vi "Gui_Prrod_Cons.vi"() -> ()   [LabVIEW 2023]
uses:
  EnumTypeDef.ctl
  <vilib>/vision/Image Controls.llb/IMAQ Image.ctl
  Control 3.ctl
  Cluster1TypeDef.ctl
panel:
  out "Image":T1(plugin-control)
  in  "OK Button":bool
  in  "File Path":path
  in  "skala szaroœci 2":u8(slide) scale=0.0..100.0
  out "Image2":T1(plugin-control)
  in  "error in (no error) 2":errorcluster
  in  "error in (no error)":errorcluster
  in  "STOP":bool
  in  "START":bool
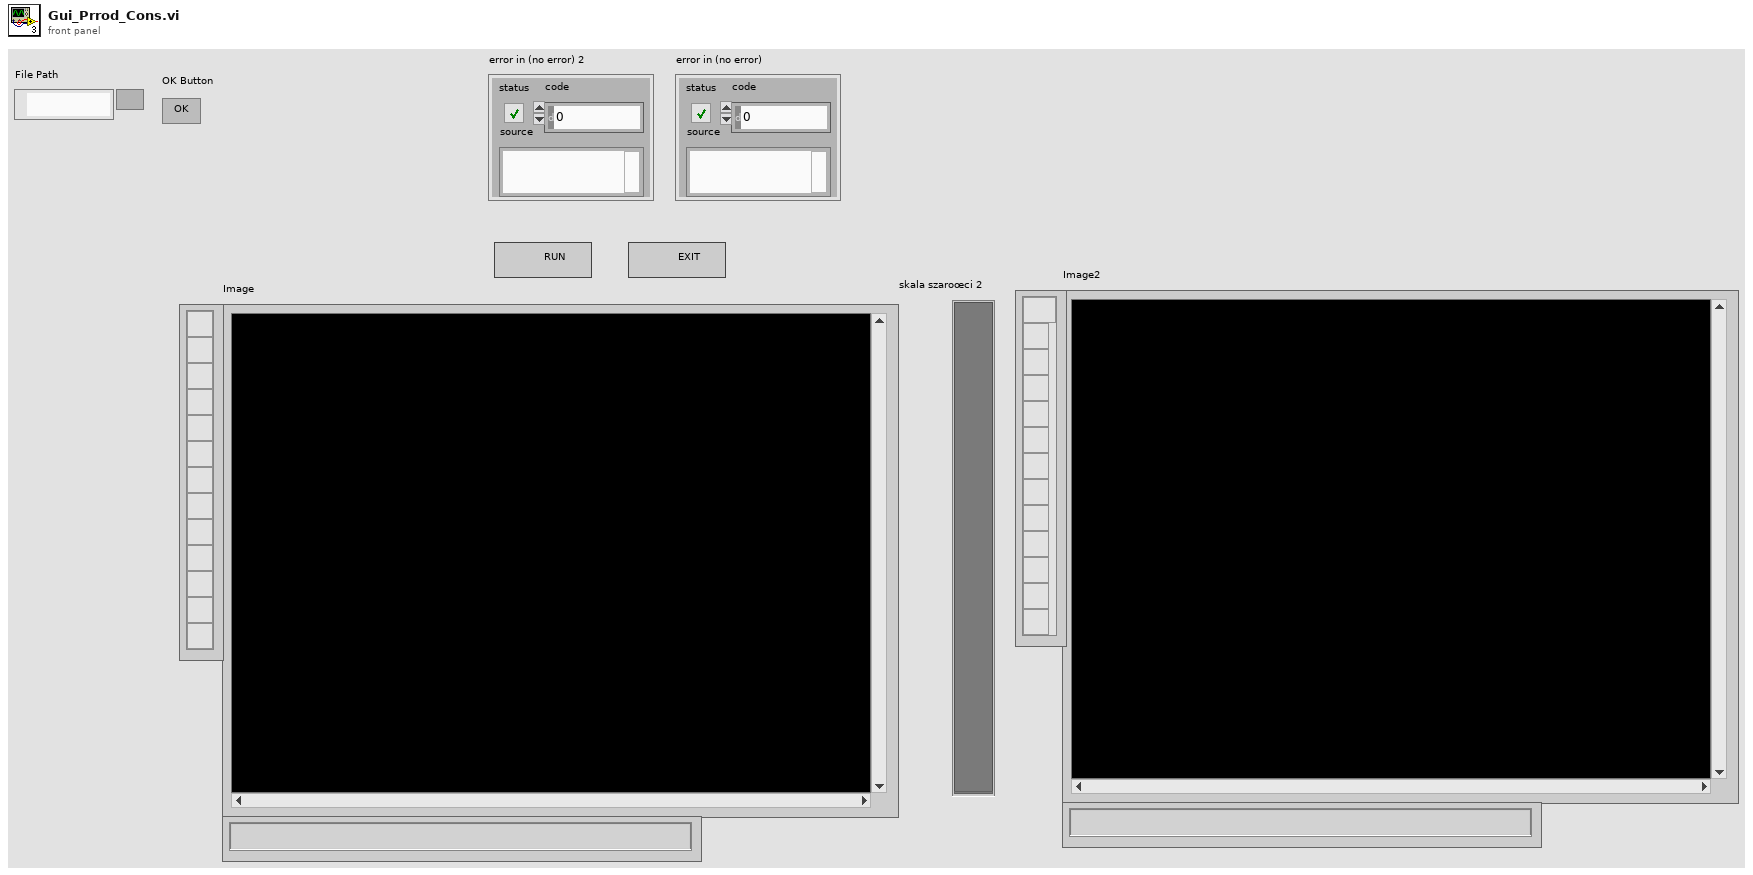
[diagram p1: front panel]
types:
  T1 = typedef "IMAQ Image.ctl" = refnum<image>
  T2 = typedef "Cluster1TypeDef.ctl" = cluster{"EditedImage":T1, "Enum":T3, "skala szaroœci 2":u8, "Data":variant, "Data2":variant}
  T3 = typedef "Control 3.ctl" = enum16{"Default", "PathLoaded", "RawImageLoaded", "LoadFile", "EditImage", "ImageEdited", "CloseAll"}
  T4 = cluster{"skala szaroœci 2":u8, "EditedImage":T1, "RawImage":T1, "Data":variant}
  T5 = typedef "EnumTypeDef.ctl" = enum16{"Initialize", "FilePathLoaded", "DisplayRaw", "EditImage", "ShutDown"}
  T6 = cluster{"skala szaroœci 2":u8, "Enum":T5, "RawImage":T1, "Data":variant}
  T7 = cluster{"EditedImage":T1, "Enum":T3, "skala szaroœci 2":u8, "Data":variant, "Data2":variant}
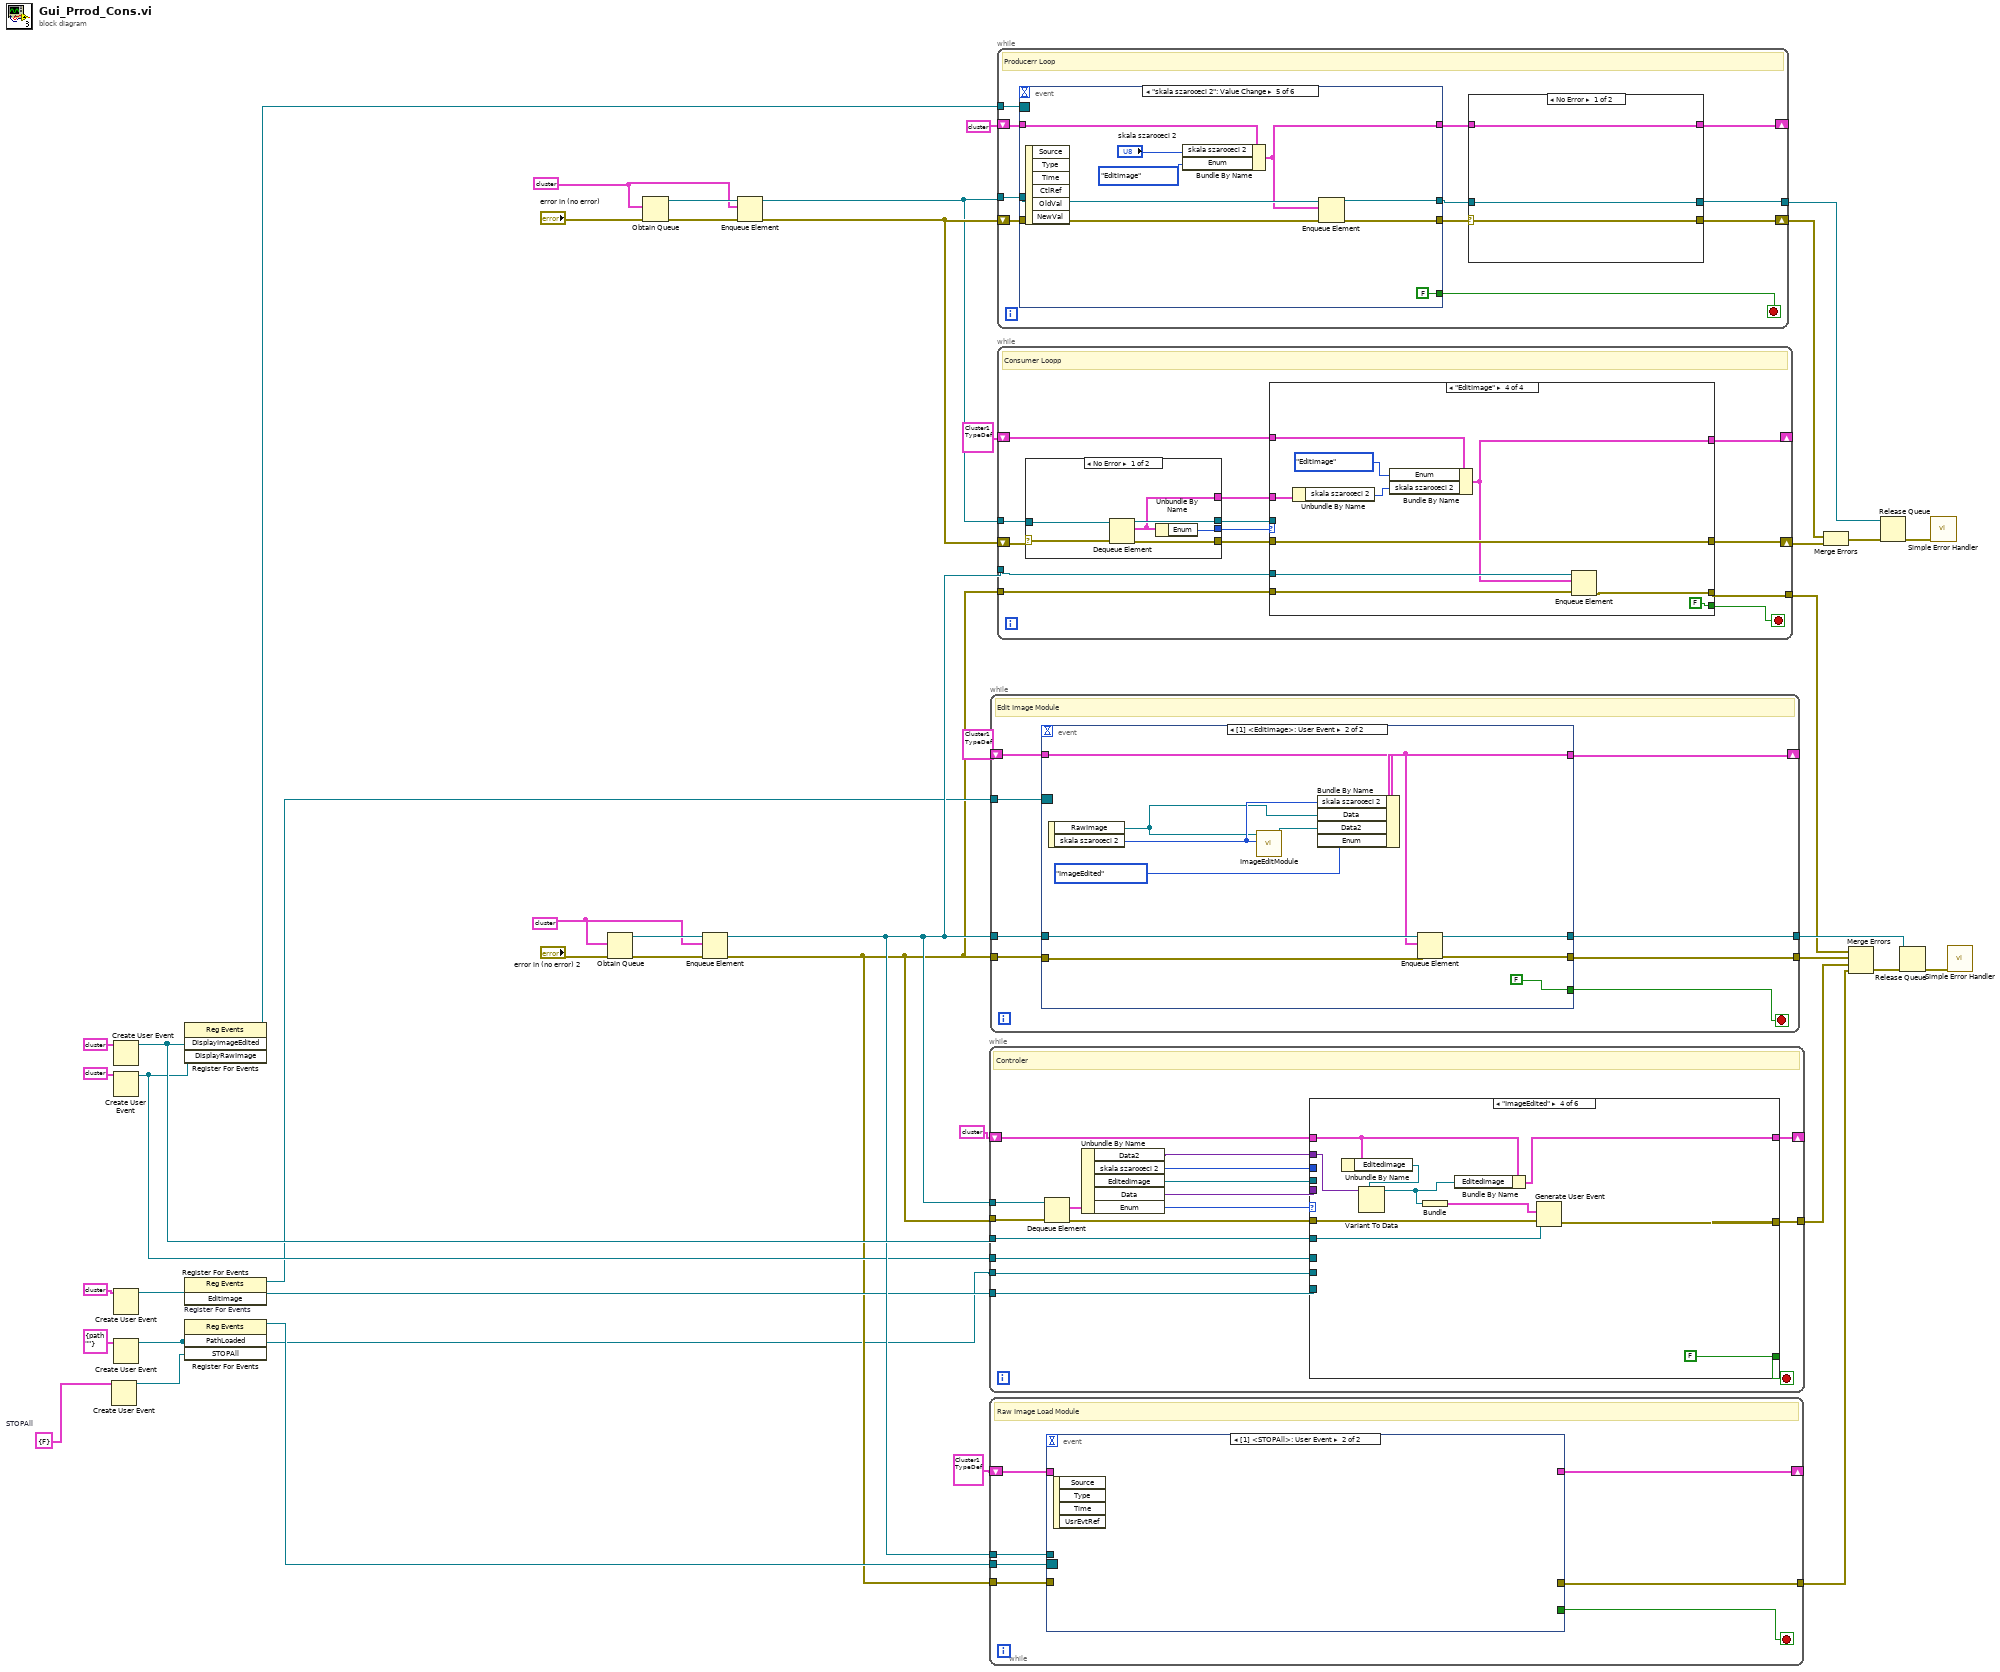
[diagram p0: block diagram]
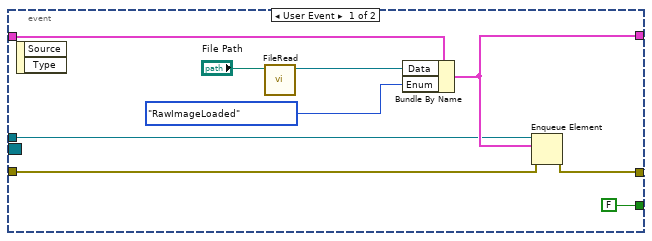
[diagram p2: hidden frame]
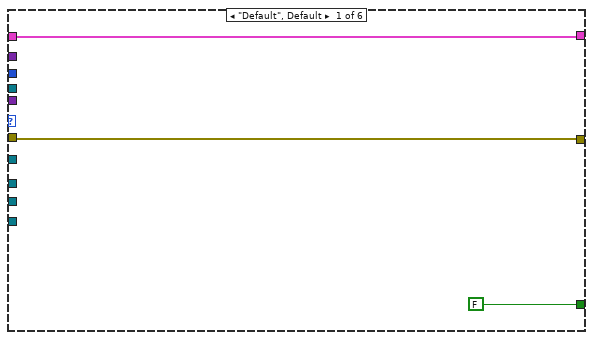
[diagram p3: hidden frame]
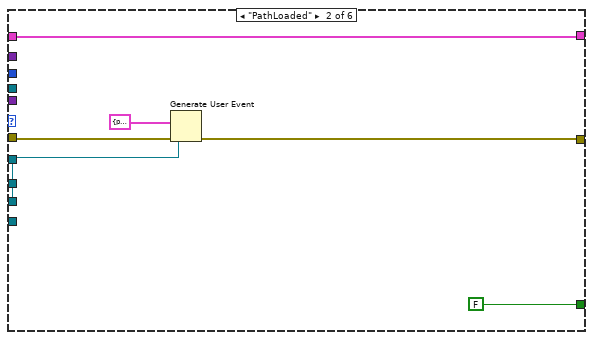
[diagram p4: hidden frame]
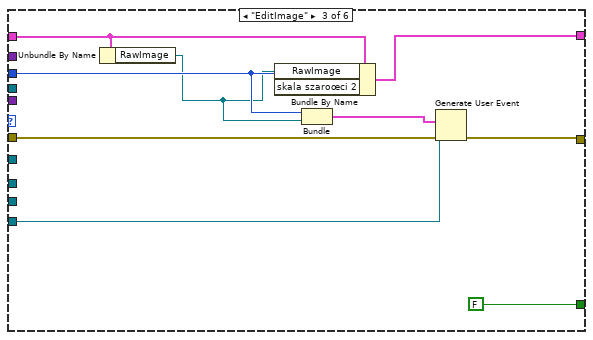
[diagram p5: hidden frame]
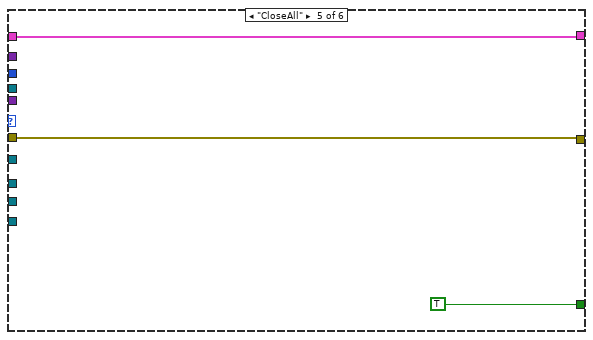
[diagram p6: hidden frame]
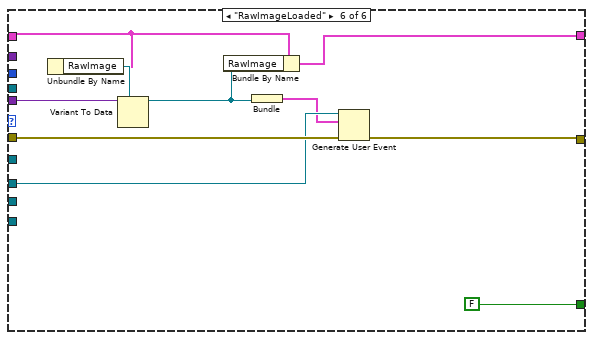
[diagram p7: hidden frame]
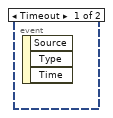
[diagram p8: hidden frame]
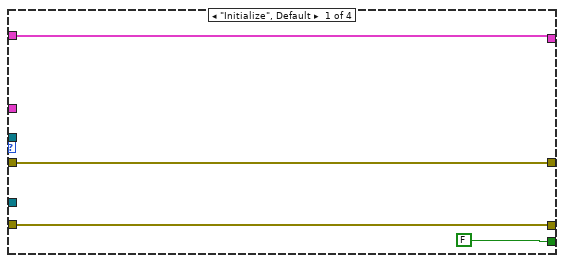
[diagram p9: hidden frame]
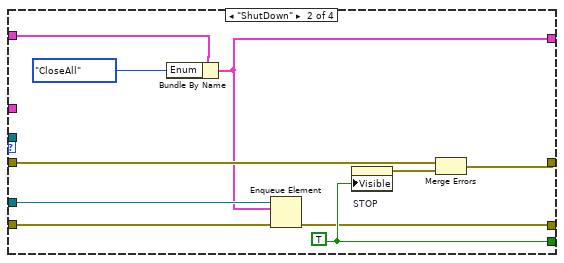
[diagram p10: hidden frame]
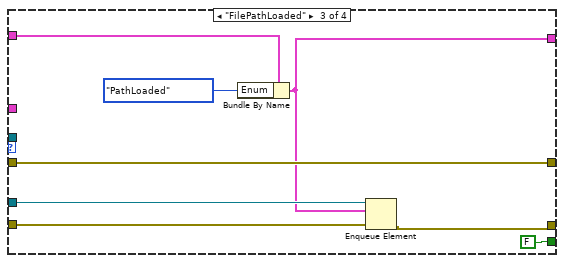
[diagram p11: hidden frame]
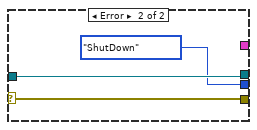
[diagram p12: hidden frame]
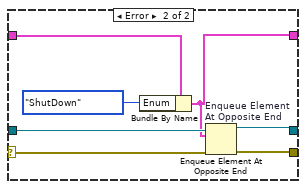
[diagram p13: hidden frame]
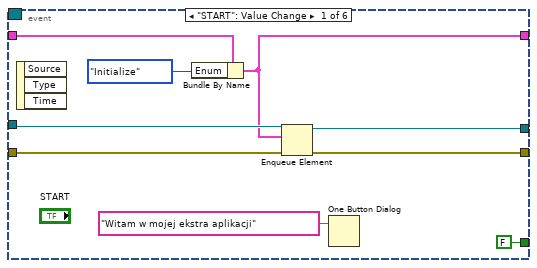
[diagram p14: hidden frame]
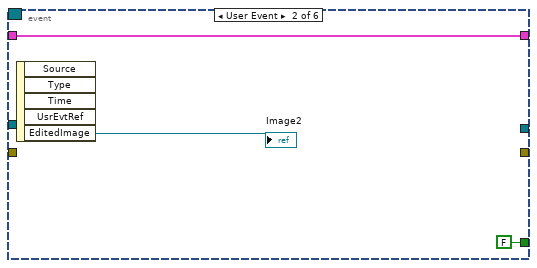
[diagram p15: hidden frame]
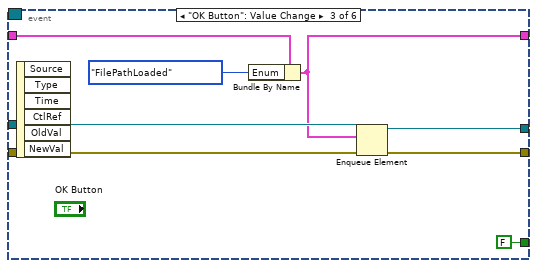
[diagram p16: hidden frame]
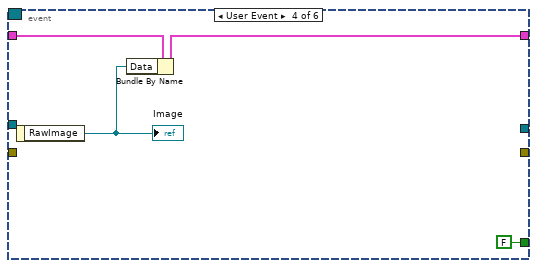
[diagram p17: hidden frame]
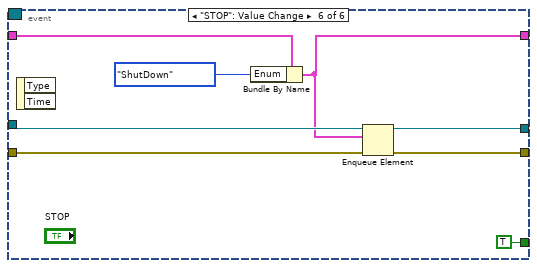
[diagram p18: hidden frame]
diagram:
  w2 = cluster{bool} {FALSE}  # STOPAll
  w16 = T6 {"skala szaroœci 2"=0, "Enum"=enum."Initialize", "RawImage"=refnum, "Data"=variant(refnum<image> refnum)} ("clusterSimple")
  w28 = T7 {"EditedImage"=refnum, "Enum"=enum."Default", "skala szaroœci 2"=0, "Data"=variant, "Data2"=variant(refnum<image> refnum)}
  n1 = Create User Event(user event datatype=w2) -> (user event=w1:refnum<user-event>)  [unwired: 1 in, 1 out]
  n2 = Create User Event(user event datatype=cluster{"EditedImage":T1} {"EditedImage"=refnum} ("DisplayImageEdited")) -> (user event=w25:refnum<user-event>)  [unwired: 1 in, 1 out]
  n3 = Create User Event(user event datatype=cluster{"RawImage":T1} {"RawImage"=refnum} ("DisplayRawImage")) -> (user event=w17:refnum<user-event>)  [unwired: 1 in, 1 out]
  n4 = Create User Event(user event datatype=cluster{"skala szaroœci 2":u8, "RawImage":T1} {"skala szaroœci 2"=0, "RawImage"=refnum} ("EditImage")) -> (user event=w13:refnum<user-event>)  [unwired: 1 in, 1 out]
  n5 = Create User Event(user event datatype=cluster{"File Path":path} {"File Path"=path ""} ("PathLoaded")) -> (user event=w7:refnum<user-event>)  [unwired: 1 in, 1 out]
  n6 = register-events(w25, w17) -> (reference out=w26:refnum<event-registration>)  [unwired: 2 in, 1 out]
  n7 = register-events(w13) -> (reference out=w10:refnum<event-registration>)  [unwired: 2 in, 1 out]
  n8 = register-events "Register For Events"(w7, w1) -> (reference out=w19:refnum<event-registration>)  [unwired: 2 in, 1 out]
  n9 = Obtain Queue(element data type=w28, error in (no error)="error in (no error) 2") -> (queue out=w30:refnum<queue>, error out=w31:errorcluster)  [unwired: 3 in, 1 out]
  n10 = Obtain Queue(element data type=w16, error in (no error)="error in (no error)") -> (queue out=w41:refnum<queue>, error out=w42:errorcluster)  [unwired: 3 in, 1 out]
  n11 = Enqueue Element(queue=w30, element=w28, error in (no error)=w31) -> (queue out=w18:refnum<queue>, error out=w9:errorcluster)  [unwired: 1 in, 1 out]
  n12 = Enqueue Element(queue=w41, element=w16, error in (no error)=w42) -> (queue out=w38:refnum<queue>, error out=w39:errorcluster)  [unwired: 1 in, 1 out]
  n13 = while {
    tunnel: w18 -> [w51]
    tunnel: w9 -> [w59]
    tunnel: w25 -> [w56]
    shift-right: [w54] -> _
    shift-left: T4 {"skala szaroœci 2"=0, "EditedImage"=refnum, "RawImage"=refnum, "Data"=variant(refnum<image> refnum)} ("EditImage") -> [w55]
    tunnel: [w52] -> w23
    tunnel: w7 -> [w50]
    tunnel: w17 -> [w49]
    tunnel: w13 -> [w48]
    stop <- w43 stop-if-true
    # "Controler"
    n14 = Dequeue Element(queue=w51, error in (no error)=w59) -> (element=w57:T7, error out=w53:errorcluster)  [unwired: 1 in, 2 out]
    n15 = Unbundle By Name(w57) -> ("Data2"=w44:variant, "skala szaroœci 2"=w45:u8, "EditedImage"=w46:T1, "Data"=w47:variant, "Enum"=w58:T3)
    n16 = case shown="\"ImageEdited\"" w58 {
      tunnel: w46 -> [_ _ _ _ _ _]
      tunnel: w56 -> [_ _ _ w87 _ _]
      tunnel: w55 -> [w62 w68 w71 w83 w88 w95]
      tunnel: [w62 w68 w74 w84 w88 w94] -> w54
      tunnel: w53 -> [w61 w67 w77 w86 w89 w100]
      tunnel: [w61 w66 w76 w85 w89 w99] -> w52
      tunnel: w50 -> [_ w65 _ _ _ _]
      tunnel: w49 -> [_ _ _ _ _ w98]
      tunnel: w48 -> [_ _ w75 _ _ _]
      tunnel: w47 -> [_ _ _ _ _ w97]
      tunnel: w45 -> [_ _ w73 _ _ _]
      tunnel: w44 -> [_ _ _ w79 _ _]
      tunnel: [FALSE FALSE FALSE FALSE TRUE FALSE] -> w43
      frame "Default", Default {
      }
      frame "PathLoaded" {
        n17 = Generate User Event(user event=w65, event data cluster=cluster{"File Path":path} {"File Path"=path ""} ("event data"), error in=w67) -> (error out=w66:errorcluster)  [unwired: 1 in, 1 out]
      }
      frame "EditImage" {
        n18 = Unbundle By Name(w71) -> ("RawImage"=w70:T1)
        n19 = Bundle By Name(cluster=w71, "RawImage"=w70, "skala szaroœci 2"=w73) -> (w74:T4)
        n20 = Bundle("skala szaroœci 2"=w73, "RawImage"=w70) -> (w72:cluster{"skala szaroœci 2":u8, "RawImage":T1})  [unwired: 1 in]
        n21 = Generate User Event(user event=w75, event data cluster=w72, error in=w77) -> (error out=w76:errorcluster)  [unwired: 1 in, 1 out]
      }
      frame "ImageEdited" {
        n22 = Unbundle By Name(w83) -> ("EditedImage"=w82:T1)
        n23 = Variant To Data(type=w82, Variant=w79) -> (data=w81:T1)  [unwired: 1 in, 1 out]
        n24 = Bundle("EditedImage"=w81) -> (w80:cluster{"EditedImage":T1})  [unwired: 1 in]
        n25 = Bundle By Name(cluster=w83, "EditedImage"=w81) -> (w84:T4)
        n26 = Generate User Event(user event=w87, event data cluster=w80, error in=w86) -> (error out=w85:errorcluster)  [unwired: 1 in, 1 out]
      }
      frame "CloseAll" {
      }
      frame "RawImageLoaded" {
        n27 = Unbundle By Name(w95) -> ("RawImage"=w96:T1)
        n28 = Variant To Data(type=w96, Variant=w97) -> (data=w93:T1)  [unwired: 1 in, 1 out]
        n29 = Bundle By Name(cluster=w95, "RawImage"=w93) -> (w94:T4)
        n30 = Bundle("RawImage"=w93) -> (w92:cluster{"RawImage":T1})  [unwired: 1 in]
        n31 = Generate User Event(user event=w98, event data cluster=w92, error in=w100) -> (error out=w99:errorcluster)  [unwired: 1 in, 1 out]
      }
    }
  }
  n32 = while {
    shift-right: [w102] -> _
    shift-left: T2 {"EditedImage"=refnum, "Enum"=enum."Default", "skala szaroœci 2"=0, "Data"=variant(refnum<image> refnum), "Data2"=variant(refnum<image> refnum)} ("Cluster") -> [w107]
    tunnel: w19 -> [w106]
    tunnel: w18 -> [w105]
    tunnel: w9 -> [w104]
    tunnel: [w103] -> w8
    stop <- w101 stop-if-true
    # "Raw Image Load Module"
    n33 = event shown="[1] <STOPAll>: User Event" {
      selector: w106 -> [_ _]
      dyn-events: _ -> [_ _]
      timeout: _ -> [_ _]
      tunnel: [w113 _] -> w102
      tunnel: w107 -> [w115 _]
      tunnel: w105 -> [w111 _]
      tunnel: w104 -> [w112 _]
      tunnel: [w110 _] -> w103
      tunnel: [FALSE _] -> w101
      event User Event {
        n34 = event-data() -> ()  [unwired: 1 in, 2 out]
        n35 = call "FileRead.vi"("File Path"="File Path") -> ("Image"=w109:T1)  [unwired: 10 in]
        n36 = Bundle By Name(cluster=w115, "Data"=w109, "Enum"=Control_3."RawImageLoaded") -> (w113:T2)
        n37 = Enqueue Element(queue=w111, element=w113, error in (no error)=w112) -> (error out=w110:errorcluster)  [unwired: 1 in, 2 out]
      }
      event User Event {
        n38 = event-data() -> ()  [unwired: 1 in, 4 out]
      }
    }
  }
  n39 = while {
    shift-right: [w120] -> _
    shift-left: T2 {"EditedImage"=refnum, "Enum"=enum."Default", "skala szaroœci 2"=0, "Data"=variant(refnum<image> refnum), "Data2"=variant(refnum<image> refnum)} ("Cluster") -> [w121]
    tunnel: [w119] -> w32
    tunnel: w18 -> [w123]
    tunnel: w9 -> [w122]
    tunnel: [w118] -> w24
    tunnel: w10 -> [w124]
    stop <- w117 stop-if-true
    # "Edit Image Module"
    n40 = event shown="[1] <EditImage>: User Event" {
      selector: w124 -> [_ _]
      dyn-events: _ -> [_ _]
      timeout: _ -> [_ _]
      tunnel: w123 -> [_ w133]
      tunnel: w122 -> [_ w132]
      tunnel: w121 -> [_ w128]
      tunnel: [_ w131] -> w120
      tunnel: [_ w130] -> w119
      tunnel: [_ w129] -> w118
      tunnel: [_ FALSE] -> w117
      event Timeout {
        n41 = event-data() -> ()  [unwired: 1 in, 3 out]
      }
      event User Event {
        n42 = event-data() -> ("RawImage"=w126:T1, "skala szaroœci 2"=w127:u8)  [unwired: 1 in]
        n43 = call "ImageEditModule.vi"("skala szaroœci 2"=w127, "New Image"=w126) -> ("Image 4"=w134:T1)  [unwired: 9 in]
        n44 = Bundle By Name(cluster=w128, "skala szaroœci 2"=w127, "Data"=w126, "Data2"=w134, "Enum"=Control_3."ImageEdited") -> (w131:T2)
        n45 = Enqueue Element(queue=w133, element=w131, error in (no error)=w132) -> (queue out=w130:refnum<queue>, error out=w129:errorcluster)  [unwired: 1 in, 1 out]
      }
    }
  }
  n46 = while {
    shift-right: [w140] -> w37
    shift-left: w39 -> [w145]
    tunnel: w38 -> [w143]
    tunnel: [w141] -> w40
    tunnel: w26 -> [w139]
    shift-right: [w136] -> _
    shift-left: T6 {"skala szaroœci 2"=0, "Enum"=enum."Initialize", "RawImage"=refnum, "Data"=variant(refnum<image> refnum)} ("clusterSimple") -> [w138]
    stop <- w146 stop-if-true
    # "Producerr Loop"
    n47 = event shown="[4] \"skala szaroœci 2\": Value Change" {
      selector: w139 -> [_ _ _ _ _ _]
      dyn-events: _ -> [_ _ _ _ _ _]
      timeout: _ -> [_ _ _ _ _ _]
      tunnel: [FALSE ("STOP") FALSE ("STOP") FALSE ("STOP") FALSE ("STOP") FALSE ("STOP") TRUE ("STOP")] -> w146
      tunnel: w145 -> [w164 _ w175 _ w184 w197]
      tunnel: [w163 _ w173 _ w186 w196] -> w144
      tunnel: w143 -> [w162 _ w176 _ w183 w195]
      tunnel: [w161 _ w174 _ w185 w194] -> w142
      tunnel: w138 -> [w160 w167 w172 w180 w188 w192]
      tunnel: [w158 w167 w170 w179 w182 w190] -> w137
      event "START": Value Change {
        n48 = event-data() -> ()  [unwired: 1 in, 3 out]
        n49 = Bundle By Name(cluster=w160, "Enum"=EnumTypeDef."Initialize") -> (w158:T6)
        n50 = Enqueue Element(queue=w162, element=w158, error in (no error)=w164) -> (queue out=w161:refnum<queue>, error out=w163:errorcluster)  [unwired: 1 in, 1 out]
        n51 = One Button Dialog(message="Witam w mojej ekstra aplikacji") -> ()  [unwired: 1 in, 1 out]
      }
      event User Event {
        n52 = event-data() -> ("EditedImage"=→"Image2":T1)  [unwired: 1 in, 4 out]
      }
      event "OK Button": Value Change {
        n53 = event-data() -> ()  [unwired: 1 in, 6 out]
        n54 = Bundle By Name(cluster=w172, "Enum"=EnumTypeDef."FilePathLoaded" ("element")) -> (w170:T6)
        n55 = Enqueue Element(queue=w176, element=w170, error in (no error)=w175) -> (queue out=w174:refnum<queue>, error out=w173:errorcluster)  [unwired: 1 in, 1 out]
      }
      event User Event {
        n56 = event-data() -> ("RawImage"=w177:T1)  [unwired: 1 in]
        "Image" <- w177
        n57 = Bundle By Name(cluster=w180, "Data"=w177) -> (w179:T6)
      }
      event "skala szaroœci 2": Value Change {
        n58 = event-data() -> ()  [unwired: 1 in, 6 out]
        n59 = Bundle By Name(cluster=w188, "skala szaroœci 2"="skala szaroœci 2", "Enum"=EnumTypeDef."EditImage") -> (w182:T6)
        n60 = Enqueue Element(queue=w183, element=w182, error in (no error)=w184) -> (queue out=w185:refnum<queue>, error out=w186:errorcluster)  [unwired: 1 in, 1 out]
      }
      event "STOP": Value Change {
        n61 = event-data() -> ()  [unwired: 1 in, 2 out]
        n62 = Bundle By Name(cluster=w192, "Enum"=EnumTypeDef."ShutDown") -> (w190:T6)
        n63 = Enqueue Element(queue=w195, element=w190, error in (no error)=w197) -> (queue out=w194:refnum<queue>, error out=w196:errorcluster)  [unwired: 1 in, 1 out]
      }
    }
    n64 = case shown="No Error" w144 {
      selector: w144 -> [w148 w156]
      tunnel: [w149 w153] -> w141
      tunnel: w142 -> [w149 w154]
      tunnel: [w148 w155] -> w140
      tunnel: w137 -> [w147 w151]
      tunnel: [w147 w150] -> w136
      frame No Error {
      }
      frame Error {
        n65 = Bundle By Name(cluster=w151, "Enum"=EnumTypeDef."ShutDown") -> (w150:T6)
        n66 = Enqueue Element At Opposite End "Enqueue Element \nAt Opposite End"(queue=w154, element=w150, error in (no error)=w156) -> (queue out=w153:refnum<queue>, error out=w155:errorcluster)  [unwired: 1 in, 1 out]
      }
    }
  }
  n67 = while {
    shift-right: [w206] -> w36
    shift-left: w39 -> [w210]
    tunnel: w38 -> [w209]
    tunnel: w18 -> [w204]
    tunnel: w9 -> [w203]
    tunnel: [w202] -> w21
    shift-right: [w200] -> _
    shift-left: T2 {"EditedImage"=refnum, "Enum"=enum."Default", "skala szaroœci 2"=0, "Data"=variant(refnum<image> refnum), "Data2"=variant(refnum<image> refnum)} ("Cluster") -> [w201]
    stop <- w198 stop-if-true
    # "Consumer Loopp"
    n68 = case shown="No Error" w210 {
      selector: w210 -> [w248 w251]
      tunnel: w209 -> [w246 w250]
      tunnel: [w247 w251] -> w207
      tunnel: [w245 w250] -> w205
      tunnel: [w244 EnumTypeDef."ShutDown" ("Enum")] -> w208
      tunnel: [w243 _] -> w199
      frame No Error {
        n69 = Dequeue Element(queue=w246, error in (no error)=w248) -> (queue out=w245:refnum<queue>, element=w243:T6, error out=w247:errorcluster)  [unwired: 1 in, 1 out]
        n70 = Unbundle By Name(w243) -> ("Enum"=w244:T5)
      }
      frame Error {
      }
    }
    n71 = case shown="\"EditImage\"" w208 {
      tunnel: w207 -> [w214 w224 w227 w237]
      tunnel: [w214 w223 w227 w237] -> w206
      tunnel: w205 -> [_ _ _ _]
      tunnel: [FALSE w221 FALSE FALSE] -> w198
      tunnel: w204 -> [_ w216 w232 w242]
      tunnel: w203 -> [w211 w218 w231 w241]
      tunnel: [w211 w217 w230 w240] -> w202
      tunnel: w201 -> [w212 w219 w228 w238]
      tunnel: [w212 w215 w225 w235] -> w200
      tunnel: w199 -> [_ _ _ w234]
      frame "Initialize", Default {
      }
      frame "ShutDown" {
        w221 = TRUE
        n72 = Bundle By Name(cluster=w219, "Enum"=Control_3."CloseAll") -> (w215:T2)
        n73 = Enqueue Element(queue=w216, element=w215, error in (no error)=w218) -> (error out=w217:errorcluster)  [unwired: 1 in, 2 out]
        n74 = property on="STOP" class="Bool"("Visible"=w221) -> (error out=w222:errorcluster)  [unwired: 2 in, 1 out]
        n75 = Merge Errors(w224, w222) -> (w223:errorcluster)
      }
      frame "FilePathLoaded" {
        n76 = Bundle By Name(cluster=w228, "Enum"=Control_3."PathLoaded") -> (w225:T2)
        n77 = Enqueue Element(queue=w232, element=w225, error in (no error)=w231) -> (error out=w230:errorcluster)  [unwired: 1 in, 2 out]
      }
      frame "EditImage" {
        n78 = Unbundle By Name(w234) -> ("skala szaroœci 2"=w233:u8)
        n79 = Bundle By Name(cluster=w238, "Enum"=Control_3."EditImage", "skala szaroœci 2"=w233) -> (w235:T2)
        n80 = Enqueue Element(queue=w242, element=w235, error in (no error)=w241) -> (error out=w240:errorcluster)  [unwired: 1 in, 2 out]
      }
    }
  }
  n81 = Merge Errors(w37, w36) -> (w35:errorcluster)
  n82 = Merge Errors(w21, w24, w23, w8) -> (w22:errorcluster)
  n83 = Release Queue(queue=w40, error in (no error)=w35) -> (error out=w33:errorcluster)  [unwired: 1 in, 2 out]
  n84 = Release Queue(queue=w32, error in (no error)=w22) -> (error out=w27:errorcluster)  [unwired: 1 in, 2 out]
  n85 = call <vilib>:"Simple Error Handler.vi"("error in (no error)"=w33) -> ()  [unwired: 4 in, 5 out]
  n86 = call <vilib>:"Simple Error Handler.vi"("error in (no error)"=w27) -> ()  [unwired: 4 in, 5 out]
